vi "ApplyMaxKernal.vi"(8 "Radius(2mm)":dbl=2.0 format="%#_13g", 9 "Z":dbl[](array[numeric]), 10 "Y":dbl[](array[numeric]), 11 "X":dbl[](array[numeric])) -> (1 "ZZ":dbl[](array[numeric]))   [LabVIEW 2024]
panel:
  out "Distance":dbl
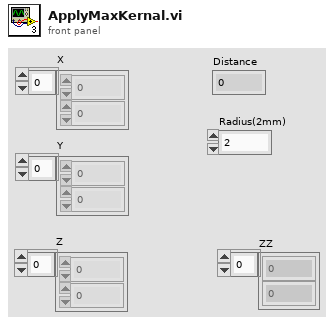
[diagram p1: front panel]
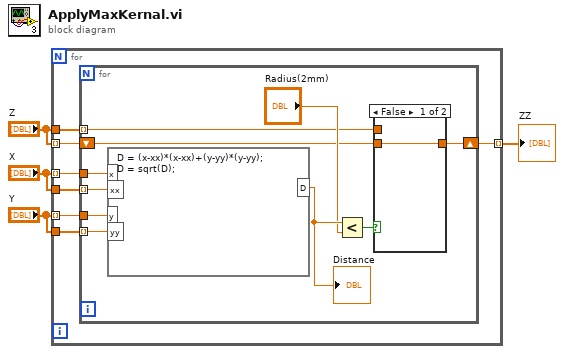
[diagram p0: block diagram]
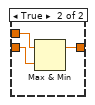
[diagram p2: hidden frame]
diagram:
  n1 = for {
    tunnel: "X" -> [w8] mode=indexing
    tunnel: "Y" -> [w7] mode=indexing
    tunnel: "Z" -> [w6] mode=indexing
    tunnel: "X" -> [w11]
    tunnel: "Y" -> [w10]
    tunnel: "Z" -> [w9]
    tunnel: [w5] -> w1 mode=indexing
    n2 = for {
      tunnel: w11 -> [w20] mode=indexing
      tunnel: w10 -> [w18] mode=indexing
      tunnel: w9 -> [w14] mode=indexing
      tunnel: w8 -> [w21]
      tunnel: w7 -> [w19]
      shift-right: [w13] -> w5
      shift-left: w6 -> [w12]
      n3 = formula code="D = (x-xx)*(x-xx)+(y-yy)*(y-yy);\nD = sqrt(D);"("x"=w21, "xx"=w20, "y"=w19, "yy"=w18) -> ("D"=w17:dbl)
      "Distance" <- w17
      n4 = Less?(x=w17, y="Radius(2mm)") -> (x < y?=w15:bool)
      n5 = case shown="False" w15 {
        tunnel: w14 -> [_ w25]
        tunnel: [w22 w23] -> w13
        tunnel: w12 -> [w22 w24]
        frame False {
        }
        frame True {
          n6 = Max & Min(x=w25, y=w24) -> (max(x,y)=w23:dbl)  [unwired: 1 out]
        }
      }
    }
  }
  "ZZ" <- w1
